vi "Initialise.vi"(8 "error in (no error)":errorcluster, 10 "Instrument Ref":string, 11 "NI Switch in":refnum<class "NI Switch.lvclass">) -> (0 "error out":errorcluster, 3 "NI Switch out":refnum<class "NI Switch.lvclass">)   [LabVIEW 2021, in "Concrete.lvlib" / "NI Switch.lvclass"]
uses:
  NI Switch.lvclass
  <instrlib>/niSwitch/niSwitch.llb/niSwitch Topologies.ctl
  NI Switch.lvclass/NI Switch.ctl
  Harware Abstraction/Switch/Switch.lvclass
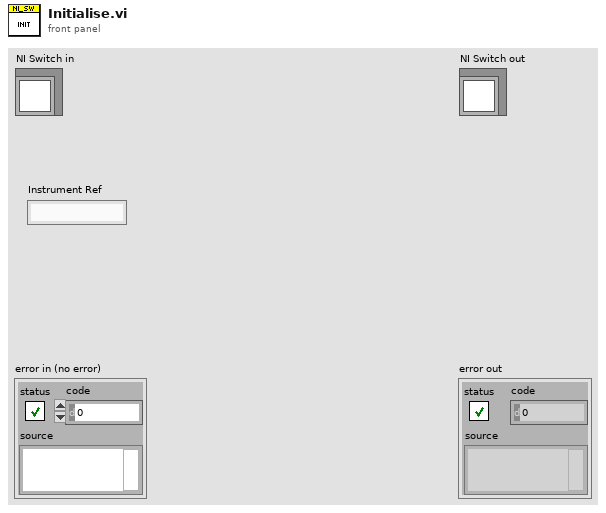
[diagram p1: front panel]
types:
  T1 = typedef "niSwitch Topologies.ctl" = string
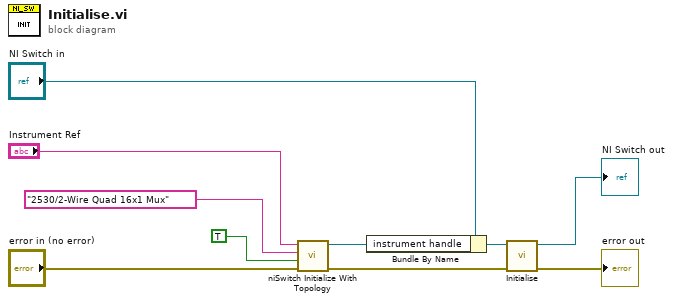
[diagram p0: block diagram]
diagram:
  n1 = call <instrlib>:"niSwitch Initialize With Topology.vi"("error in (no error)"="error in (no error)", "reset device (boolean value)"=TRUE, "topology name"=T1 "2530/2-Wire Quad 16x1 Mux", "resource name"="Instrument Ref") -> ("error out"=w6:errorcluster, "instrument handle out"=w1:refnum<k15>)  [unwired: 6 in]
  n2 = Bundle By Name(cluster="NI Switch in", "instrument handle"=w1) -> (w2:refnum<class "NI Switch.lvclass">)
  n3 = call-parent "Initialise.vi"("error in (no error)"=w6, "Instrument in"=w2) -> ("error out"=→"error out":errorcluster, "Instrument out"=→"NI Switch out":refnum<class "NI Switch.lvclass">)  [unwired: 8 in]
